vi "WFDC Setup Camera.vi"(7 "Camera Notifier Name":string) -> (4 "ROI":T1, 8 "Exp Time":dbl, 15 "Canceled?":bool)   [LabVIEW 2020]
uses:
  Device Library/Cameras/IDS/IDS Controls/IDS ROI.ctl
  Device Library/Cameras/IDS/IDS Controls/IDS Actions.ctl
  Device Library/Cameras/IDS/IDS Controls/IDS Parameters.ctl
  Device Library/Cameras/IDS/IDS Controls/IDS Parameter List.ctl
  <vilib>/Utility/miscctls.llb/LVPointTypeDef.ctl
  971de522-e521-432e-a3bb-4c971b991dd5.vi
panel:
  in  "Exposure Time (ms)":dbl=1.0
  in  "Tool Selection":enum32{"Zoom Tool", "ROI Tool", "Pan Tool"}(radio)
  in  "Cancel":bool
  in  "Done":bool
  out "Camera Display":T2(plugin-control)
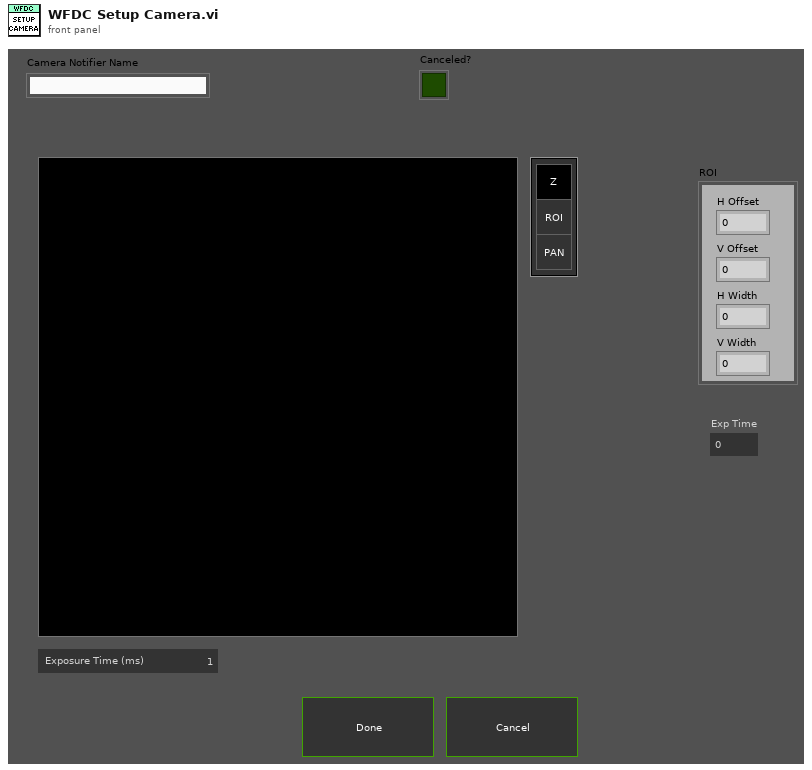
[diagram p1: front panel]
types:
  T1 = typedef "IDS ROI.ctl" = cluster{"H Offset":i32, "V Offset":i32, "H Width":i32, "V Width":i32}
  T2 = typedef "IMAQ Image.ctl" = refnum<image>
  T3 = enum16{"Always On", "Always Off", "Off While Running"}
  T4 = typedef "LVPointTypeDef.ctl" = cluster{"Horizontal":i16, "Vertical":i16}
  T5 = typedef "IDS Actions.ctl" = enum16{"Error Check", "Initialize", "Preview", "Record", "Abort", "Record Settings", "Set Parameter", "Get Parameter", "Set ROI", "Get ROI", "Status", "Quit"}
  T6 = typedef "IDS Parameters.ctl" = cluster{"Parameter":T7, "Value":dbl}
  T7 = typedef "IDS Parameter List.ctl" = enum16{"Exposure Time (s)", "Binning"}
  T8 = typedef "LVRectTypeDef.ctl" = cluster{"Left":i16, "Top":i16, "Right":i16, "Bottom":i16}
  T9 = typedef "LVBoundsTypeDef.ctl" = cluster{"Width":u32, "Height":u32}
  T10 = cluster{"Global Rectangle":i32[], "Contours":cluster{"Contour Type":u32, "ROI Type":u32, "Points":i32[]}[]}
  T11 = cluster{"Contour Type":u32, "ROI Type":u32, "Points":i32[]}[]
  T12 = cluster{"Contour Type":u32, "ROI Type":u32, "Points":i32[]}
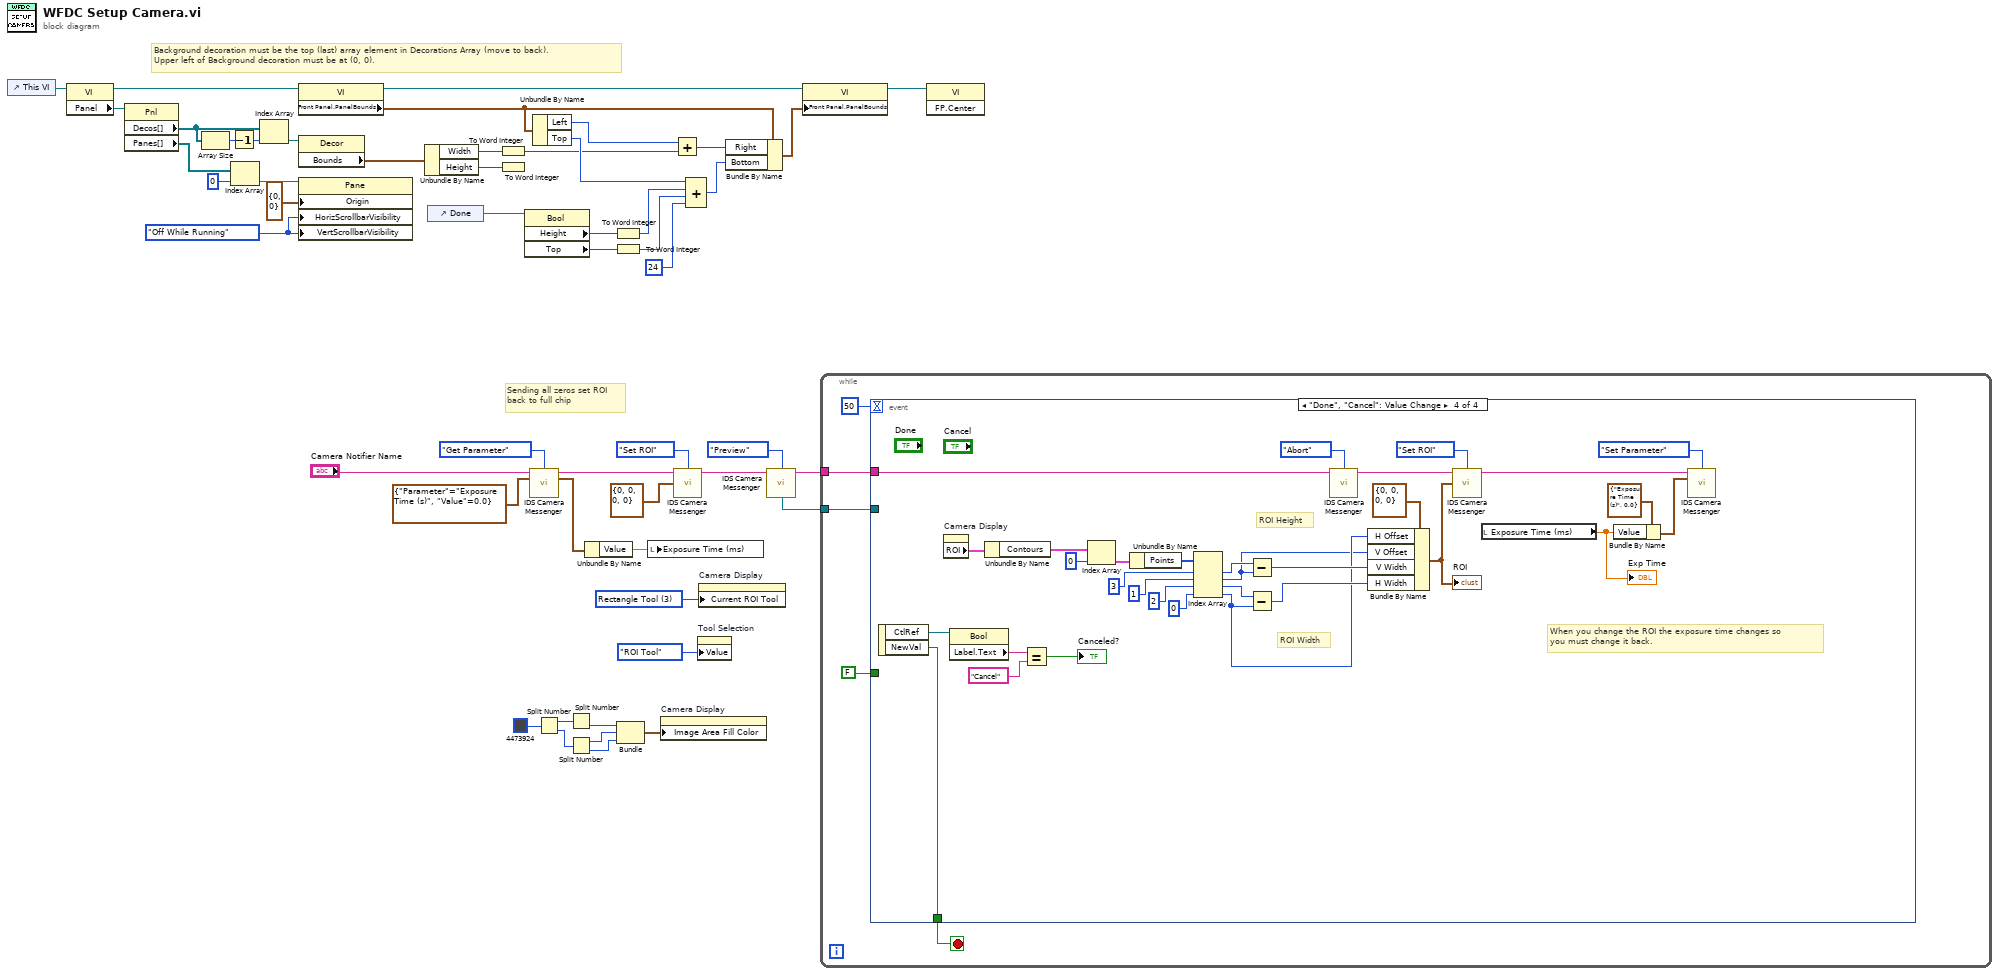
[diagram p0: block diagram]
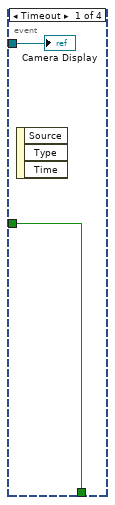
[diagram p2: hidden frame]
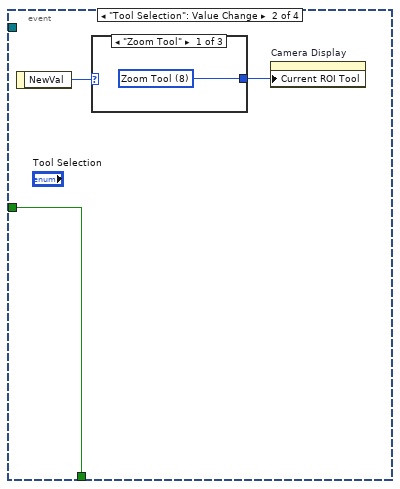
[diagram p3: hidden frame]
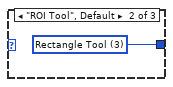
[diagram p4: hidden frame]
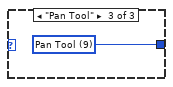
[diagram p5: hidden frame]
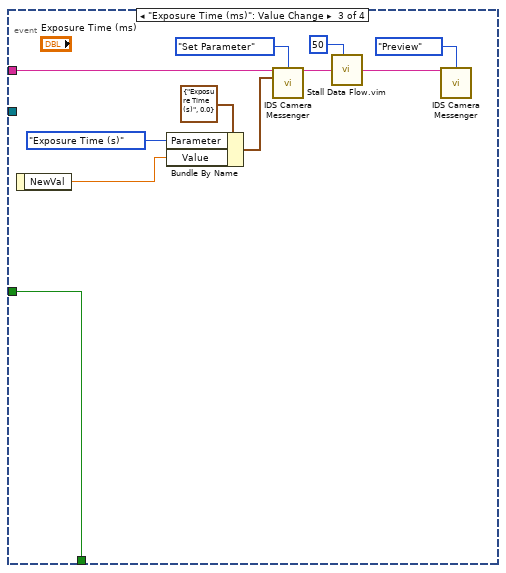
[diagram p6: hidden frame]
diagram:
  w20 = T3."Off While Running" ("Vertical Scrollbar Visibility")
  w43 = u32 3 items=["Zoom Tool"=8, "Selection Tool"=0, "Pan Tool"=9, "Point Tool"=1, "Line Tool"=2, "Rectangle Tool"=3, "Rotated Rectangle Tool"=12, "Polyline Tool"=10, "Polygon Tool"=5, "Freehand Tool"=11, "Closed Freehand Tool"=6, "Ellipse Tool"=4, "Annulus Tool"=7] ("Current ROI Tool")
  # "Background decoration must be the top (last) array element in Decorations Array (move to back).\nUpper left of Background decoration must be at (0, 0)."
  # "Sending all zeros set ROI\nback to full chip"
  n1 = control-ref of="This VI"() -> (w12:refnum<vi>)
  n2 = property class="VI"(reference=w12) -> (reference out=w21:refnum<vi>, "Panel"=w13:refnum<vi>)  [unwired: 1 in, 1 out]
  n3 = property class="Pnl"(reference=w13) -> ("Decos[]"=w11:refnum<vi>[], "Panes[]"=w17:refnum<vi>[])  [unwired: 1 in, 2 out]
  n4 = Array Size(array=w11) -> (size(s)=w9:i32)
  n5 = Decrement(x=w9) -> (x-1=w10:i32)
  n6 = Index Array(array=w17, index=0) -> (element=w16:refnum<vi>)
  n7 = Index Array(array=w11, index=w10) -> (element=w19:refnum<vi>)
  n8 = property class="VI"(reference=w21) -> (reference out=w23:refnum<vi>, "Front Panel.PanelBounds"=w24:T8)  [unwired: 1 in, 1 out]
  n9 = property class="Decor"(reference=w19) -> ("Bounds"=w22:T9)  [unwired: 1 in, 2 out]
  n10 = property class="Pane"(reference=w16, "Origin"=T4 {"Horizontal"=0, "Vertical"=0}, "HorizScrollbarVisibility"=w20, "VertScrollbarVisibility"=w20) -> ()  [unwired: 1 in, 2 out]
  n11 = Unbundle By Name(w22) -> ("Width"=w27:u32, "Height"=w30:u32)
  n12 = control-ref of="Done"() -> (w14:refnum<vi>)
  n13 = To Word Integer(number=w27) -> (16bit integer=w29:i16)
  n14 = To Word Integer(number=w30) -> ()  [unwired: 1 out]
  n15 = property class="Bool"(reference=w14) -> ("Height"=w32:u32, "Top"=w33:i32)  [unwired: 1 in, 2 out]
  n16 = call "IDS Camera Messenger.vi"("Notifier Name"="Camera Notifier Name", "IDS Actions"=IDS_Actions."Get Parameter", "IDS Parameter"=T6 {"Parameter"=enum."Exposure Time (s)", "Value"=0.0}) -> ("Notifier Name (Dup)"=w40:string, "IDS Parameter"=w45:T6)  [unwired: 7 in, 4 out]
  n17 = Unbundle By Name(w24) -> ("Left"=w26:i16, "Top"=w37:i16)
  n18 = Split Number(x=u32 4473924) -> (hi(x)=w6:u16, lo(x)=w5:u16)
  n19 = Split Number(x=w6) -> (lo(x)=w4:u8)  [unwired: 1 out]
  n20 = Split Number(x=w5) -> (hi(x)=w3:u8, lo(x)=w2:u8)
  n21 = Unbundle By Name(w45) -> ("Value"=w44:dbl)
  n22 = To Word Integer(number=w32) -> (16bit integer=w35:i16)
  n23 = To Word Integer(number=w33) -> (16bit integer=w36:i16)
  n24 = Bundle(w4, w3, w2) -> (w1:cluster{u8, u8, u8})  [unwired: 1 in]
  n25 = local write "Exposure Time (ms)"(w44) -> ()
  n26 = property on="Camera Display" class="ImageControl"("Image Area Fill Color"=w1) -> ()  [unwired: 2 in, 2 out]
  n27 = Add(x=w26, y=w29) -> (x+y=w28:i16)
  n28 = call "IDS Camera Messenger.vi"("Notifier Name"=w40, "IDS Actions"=IDS_Actions."Set ROI", "ROI Setup"=T1 {"H Offset"=0, "V Offset"=0, "H Width"=0, "V Width"=0}) -> ("Notifier Name (Dup)"=w39:string)  [unwired: 7 in, 5 out]
  n29 = Compound Arithmetic op=ADD(w37, w35, w36, i16 24 ("y")) -> (w31:i16)
  n30 = property on="Tool Selection" class="RadioBtnsControl (strict)"("Value"=enum32{"Zoom Tool", "ROI Tool", "Pan Tool"}."ROI Tool" ("Tool Selection")) -> ()  [unwired: 2 in, 2 out]
  n31 = property on="Camera Display" class="ImageControl"("Current ROI Tool"=w43) -> ()  [unwired: 2 in, 2 out]
  n32 = Bundle By Name(cluster=w24, "Right"=w28, "Bottom"=w31) -> (w25:T8)
  n33 = call "IDS Camera Messenger.vi"("Notifier Name"=w39, "IDS Actions"=IDS_Actions."Preview") -> ("Notifier Name (Dup)"=w49:string, "Image Ref"=w50:T2)  [unwired: 8 in, 4 out]
  n34 = property class="VI"(reference=w23, "Front Panel.PanelBounds"=w25) -> (reference out=w8:refnum<vi>)  [unwired: 1 in, 1 out]
  n35 = while {
    tunnel: w50 -> [w54]
    tunnel: w49 -> [w52]
    stop <- w56 stop-if-true
    n36 = event shown="[3] \"Done\", \"Cancel\": Value Change" {
      selector: _ -> [_ _ _ _]
      dyn-events: _ -> [_ _ _ _]
      timeout: 50 -> [_ _ _ _]
      tunnel: [w58 w61 w75 w103] -> w56
      tunnel: FALSE -> [w58 w61 w75 _]
      tunnel: w54 -> [w57 _ _ _]
      tunnel: w52 -> [_ _ w73 w101]
      event Timeout {
        n37 = event-data() -> ()  [unwired: 1 in, 3 out]
        "Camera Display" <- w57
      }
      event "Tool Selection": Value Change {
        n38 = event-data() -> ("NewVal"=w60:enum32{"Zoom Tool", "ROI Tool", "Pan Tool"})  [unwired: 1 in]
        n39 = case shown="\"Zoom Tool\"" w60 {
          tunnel: [w62 w63 w64] -> w59
          frame "Zoom Tool" {
            w62 = u32 8 items=["Zoom Tool"=8, "Selection Tool"=0, "Pan Tool"=9, "Point Tool"=1, "Line Tool"=2, "Rectangle Tool"=3, "Rotated Rectangle Tool"=12, "Polyline Tool"=10, "Polygon Tool"=5, "Freehand Tool"=11, "Closed Freehand Tool"=6, "Ellipse Tool"=4, "Annulus Tool"=7] ("Current ROI Tool")
          }
          frame "ROI Tool", Default {
            w63 = u32 3 items=["Zoom Tool"=8, "Selection Tool"=0, "Pan Tool"=9, "Point Tool"=1, "Line Tool"=2, "Rectangle Tool"=3, "Rotated Rectangle Tool"=12, "Polyline Tool"=10, "Polygon Tool"=5, "Freehand Tool"=11, "Closed Freehand Tool"=6, "Ellipse Tool"=4, "Annulus Tool"=7] ("Current ROI Tool")
          }
          frame "Pan Tool" {
            w64 = u32 9 items=["Zoom Tool"=8, "Selection Tool"=0, "Pan Tool"=9, "Point Tool"=1, "Line Tool"=2, "Rectangle Tool"=3, "Rotated Rectangle Tool"=12, "Polyline Tool"=10, "Polygon Tool"=5, "Freehand Tool"=11, "Closed Freehand Tool"=6, "Ellipse Tool"=4, "Annulus Tool"=7] ("Current ROI Tool")
          }
        }
        n40 = property on="Camera Display" class="ImageControl"("Current ROI Tool"=w59) -> ()  [unwired: 2 in, 2 out]
      }
      event "Exposure Time (ms)": Value Change {
        n41 = event-data() -> ("NewVal"=w69:dbl)  [unwired: 1 in]
        n42 = Bundle By Name(cluster=T6 {"Parameter"=enum."Exposure Time (s)", "Value"=0.0} ("IDS Parameter"), "Parameter"=IDS_Parameter_List."Exposure Time (s)", "Value"=w69) -> (w70:T6)
        n43 = call "IDS Camera Messenger.vi"("Notifier Name"=w73, "IDS Actions"=IDS_Actions."Set Parameter", "IDS Parameter"=w70) -> ("Notifier Name (Dup)"=w67:string)  [unwired: 7 in, 5 out]
        n44 = call "Stall Data Flow.vim"("value in"=w67, "milliseconds to wait"=u32 50) -> ("value out"=w66:string)  [unwired: 1 out]
        n45 = call "IDS Camera Messenger.vi"("Notifier Name"=w66, "IDS Actions"=IDS_Actions."Preview") -> ()  [unwired: 8 in, 6 out]
      }
      event "Done", "Cancel": Value Change {
        # "When you change the ROI the exposure time changes so\nyou must change it back."
        # "ROI Width"
        # "ROI Height"
        n46 = event-data() -> ("CtlRef"=w106:refnum<vi>, "NewVal"=w103:bool)  [unwired: 1 in]
        n47 = property on="Camera Display" class="ImageControl"() -> ("ROI"=w97:T10)  [unwired: 2 in, 2 out]
        n48 = property class="Bool"(reference=w106) -> ("Label.Text"=w105:string)  [unwired: 1 in, 2 out]
        n49 = Unbundle By Name(w97) -> ("Contours"=w96:T11)
        n50 = Equal?(x=w105, y="Cancel") -> (x = y?=→"Canceled?":bool)
        n51 = Index Array(array=w96, index=0) -> (element=w95:T12)
        n52 = Unbundle By Name(w95) -> ("Points"=w98:i32[])
        n53 = Index Array(array=w98, index #1=3 ("index"), index #2=1 ("index"), index #3=2 ("index"), index #4=0 ("index")) -> (element #1=w100:i32, element #2=w91:i32, element #3=w99:i32, element #4=w92:i32)
        n54 = Subtract(x=w100, y=w91) -> (x-y=w94:i32)
        n55 = Subtract(x=w99, y=w92) -> (x-y=w93:i32)
        n56 = call "IDS Camera Messenger.vi"("Notifier Name"=w101, "IDS Actions"=IDS_Actions."Abort") -> ("Notifier Name (Dup)"=w83:string)  [unwired: 8 in, 5 out]
        n57 = Bundle By Name(cluster=T1 {"H Offset"=0, "V Offset"=0, "H Width"=0, "V Width"=0} ("ROI Setup"), "H Offset"=w92, "V Offset"=w91, "V Width"=w94, "H Width"=w93) -> (w76:T1)
        "ROI" <- w76
        n58 = call "IDS Camera Messenger.vi"("Notifier Name"=w83, "IDS Actions"=IDS_Actions."Set ROI", "ROI Setup"=w76) -> ("Notifier Name (Dup)"=w81:string)  [unwired: 7 in, 5 out]
        n59 = local read "Exposure Time (ms)"() -> (w80:dbl)
        "Exp Time" <- w80
        n60 = Bundle By Name(cluster=T6 {"Parameter"=enum."Exposure Time (s)", "Value"=0.0} ("IDS Parameter"), "Value"=w80) -> (w78:T6)
        n61 = call "IDS Camera Messenger.vi"("Notifier Name"=w81, "IDS Actions"=IDS_Actions."Set Parameter", "IDS Parameter"=w78) -> ()  [unwired: 7 in, 6 out]
      }
    }
  }
  n62 = invoke class="VI" method="FP.Center"(reference=w8) -> ()  [unwired: 2 in, 3 out]
